vi "Update.vi"(4 "TypeMap in":refnum<class "TypeMap.lvclass">, 6 "commandTimeout":i32=-1, 8 "error in (no error)":errorcluster, 10 "object in":refnum<class>, 11 "SqlMapper in":refnum<class "SqlMapper.lvclass">) -> (0 "error out":errorcluster, 1 "affectedRows":i32, 2 "object out":refnum<class>, 3 "SqlMapper out":refnum<class "SqlMapper.lvclass">)   [LabVIEW 2020, in "ORM_API.lvlib"]
doc: "UPDATE a single entities."
uses:
  ORM_API.lvlib
  <vilib>/Viviota/shared/ORM.lvlibp/ORM/TypeMap/TypeMap.lvclass
  <vilib>/Viviota/shared/ORM.lvlibp/ORM/SqlMapper/SqlMapper.lvclass
  <userlib>/_OpenG.lib/lvdata/lvdata.llb/LVOOP Is Default Value__ogtk.vi
  <vilib>/Viviota/shared/ORM.lvlibp/ORM/TypeMap/Read TypeMap.vi
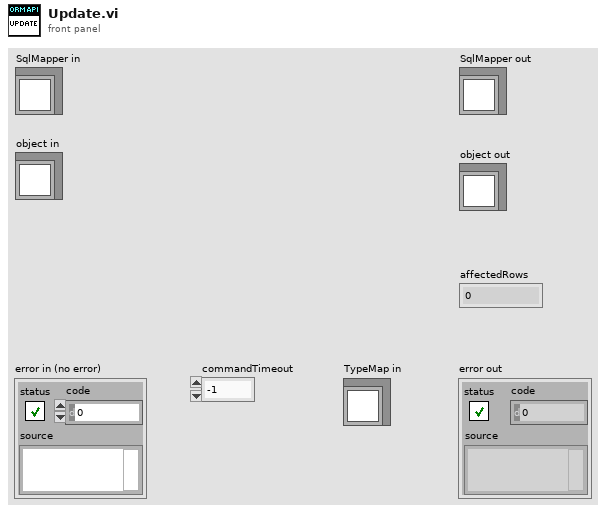
[diagram p1: front panel]
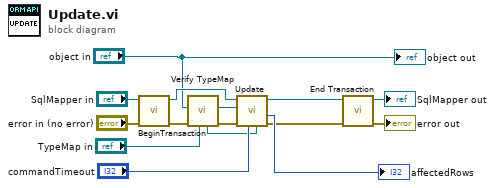
[diagram p0: block diagram]
diagram:
  n1 = call-dynamic "BeginTransaction.vi"("error in (no error)"="error in (no error)", "SqlMapper in"="SqlMapper in") -> ("error out"=w15:errorcluster, "SqlMapper out"=w8:refnum<class "SqlMapper.lvclass">)  [unwired: 8 in]
  n2 = call "Verify TypeMap.vi"("TypeMap in"="TypeMap in", "error in (no error)"=w15, "Type in"="object in") -> ("error out"=w14:errorcluster, "Type out"=w5:refnum<class>, "TypeMap out"=w4:refnum<class "TypeMap.lvclass">)  [unwired: 6 in]
  n3 = call-dynamic "Update.vi"("TypeMap in"=w4, "commandTimeout"="commandTimeout", "error in (no error)"=w14, "object in"=w5, "SqlMapper in"=w8) -> ("error out"=w2:errorcluster, "affectedRows"=→"affectedRows":i32, "SqlMapper out"=w13:refnum<class "SqlMapper.lvclass">)  [unwired: 4 in]
  n4 = call <vilib>:"End Transaction.vi"("error in (no error)"=w2, "SqlMapper in"=w13) -> ("error out"=→"error out":errorcluster, "SqlMapper out"=→"SqlMapper out":refnum<class "SqlMapper.lvclass">)  [unwired: 8 in]
  "object out" <- "object in"
